vi "AlliGator Calibrate Single Phasor Plot.vi"(0 "Raw Phasor Plot":T6={"Phasor Plot Name"="", "Raw Phasor Plot"=[], "Phasor Frequency"=160000000.0, "[Decay Metadata]"=[], "Raw Phasor Plot SDV"=[], "Phasor SDV Options"={"Compute Estimated SDV"=FALSE, "# Replicas"=100, "Use Estimated Average Phasor"=FALSE}, "[Calibration Phasor]"=[], "Intensity Array"=[]} {"[Decay Metadata]"."# Folds" min=1; "[Decay Metadata]"."ROI Descriptor"."Contours"."Type" items=["No Selection", "Point", "Line", "Rectangle", "Oval", "Polygon", "Freehand Region", "Annulus", "Unused2", "Unused3", "Broken Line", "Freehand Line", "Rotated Rectangle"]}, 5 "Calibration Phasor":T1, 7 "Calibration Phasor Series":T5, 9 "Phasor Calibration Map":T2={"Phasor Frequency"=80000000.0, "Calibration Lifetime"=1e-09, "ROI Centers"=[], "ROI Descriptors"=[], "Map Resolution X"=0, "Map Resolution Y"=0, "z Array"=[]} {"ROI Descriptors"."Contours"."Type" items=["No Selection", "Point", "Line", "Rectangle", "Oval", "Polygon", "Freehand Region", "Annulus", "Unused2", "Unused3", "Broken Line", "Freehand Line", "Rotated Rectangle"]}, 11 "Error In":errorcluster, 12 "Calibration Map MD5 Digest":string, 13 "Phasor Frequency":dbl[unit]) -> (4 "[Calibrated Phasor]":T4[](array[typedef]), 6 "# Recalibrated Phasors":i32, 8 "[Calibration Phasor]":T1[](array[typedef]), 15 "Error Out":errorcluster)   [LabVIEW 2021, in "AlliGator Phasor Calibration.lvlib"]
doc: "Applies phasor calibration to a single phasor plot.\n\nTakes into account whether a single phasor calibration, a phasor map or a phasor calibration series is used.\n\nFor a calibration map, takes into account the location of each individual phasor in the phasor plot."
uses:
  AlliGator Phasor Calibration.lvlib
  Phasor Graph/AlliGator Raw Phasor Plot Data v5.ctl
  Phasor/Phasor (g, s).ctl
  Phasor Graph/AlliGator Decay Metadata v3.ctl
  Decay Analysis/Decay Preprocessing/AlliGator Decay Background Subtraction Info.ctl
  Decay Analysis/Decay Preprocessing/AlliGator Baseline Subtraction Method.ctl
  Graphs/XY Graph/XY Graph Plot Shift Parameters.ctl
  Graphs/XY Graph/XY Graph Plot Shift Method.ctl
  Decay Analysis/Decay Preprocessing/AlliGator Decay Extrapolation Parameters.ctl
  Phasor/Phasor Standard Deviation Options.ctl
  Phasor/Calibration Phasor (m, phi).ctl
  Phasor/Phasor Reference Series.ctl
  Phasor/Phasor Calibration Map v2.ctl
  Settings/AlliGator Settings List.ctl
  Phasor/Phasor Calibration Type.ctl
  Utilities/Utilities.lvlib
  Phasor/Phasor.lvlib
  Settings/AlliGator Settings.lvlib
  Phasor Graph/AlliGator Phasor Graph.lvlib
  Decay Analysis/Decay Preprocessing/AlliGator Decay Preprocessing.lvlib
  Graphs/XY Graph/XY Graph Add-Ons.lvlib
panel:
  # "see the AlliGator License on the block diagram (Ctrl+E or Window:Show Block Diagram)"
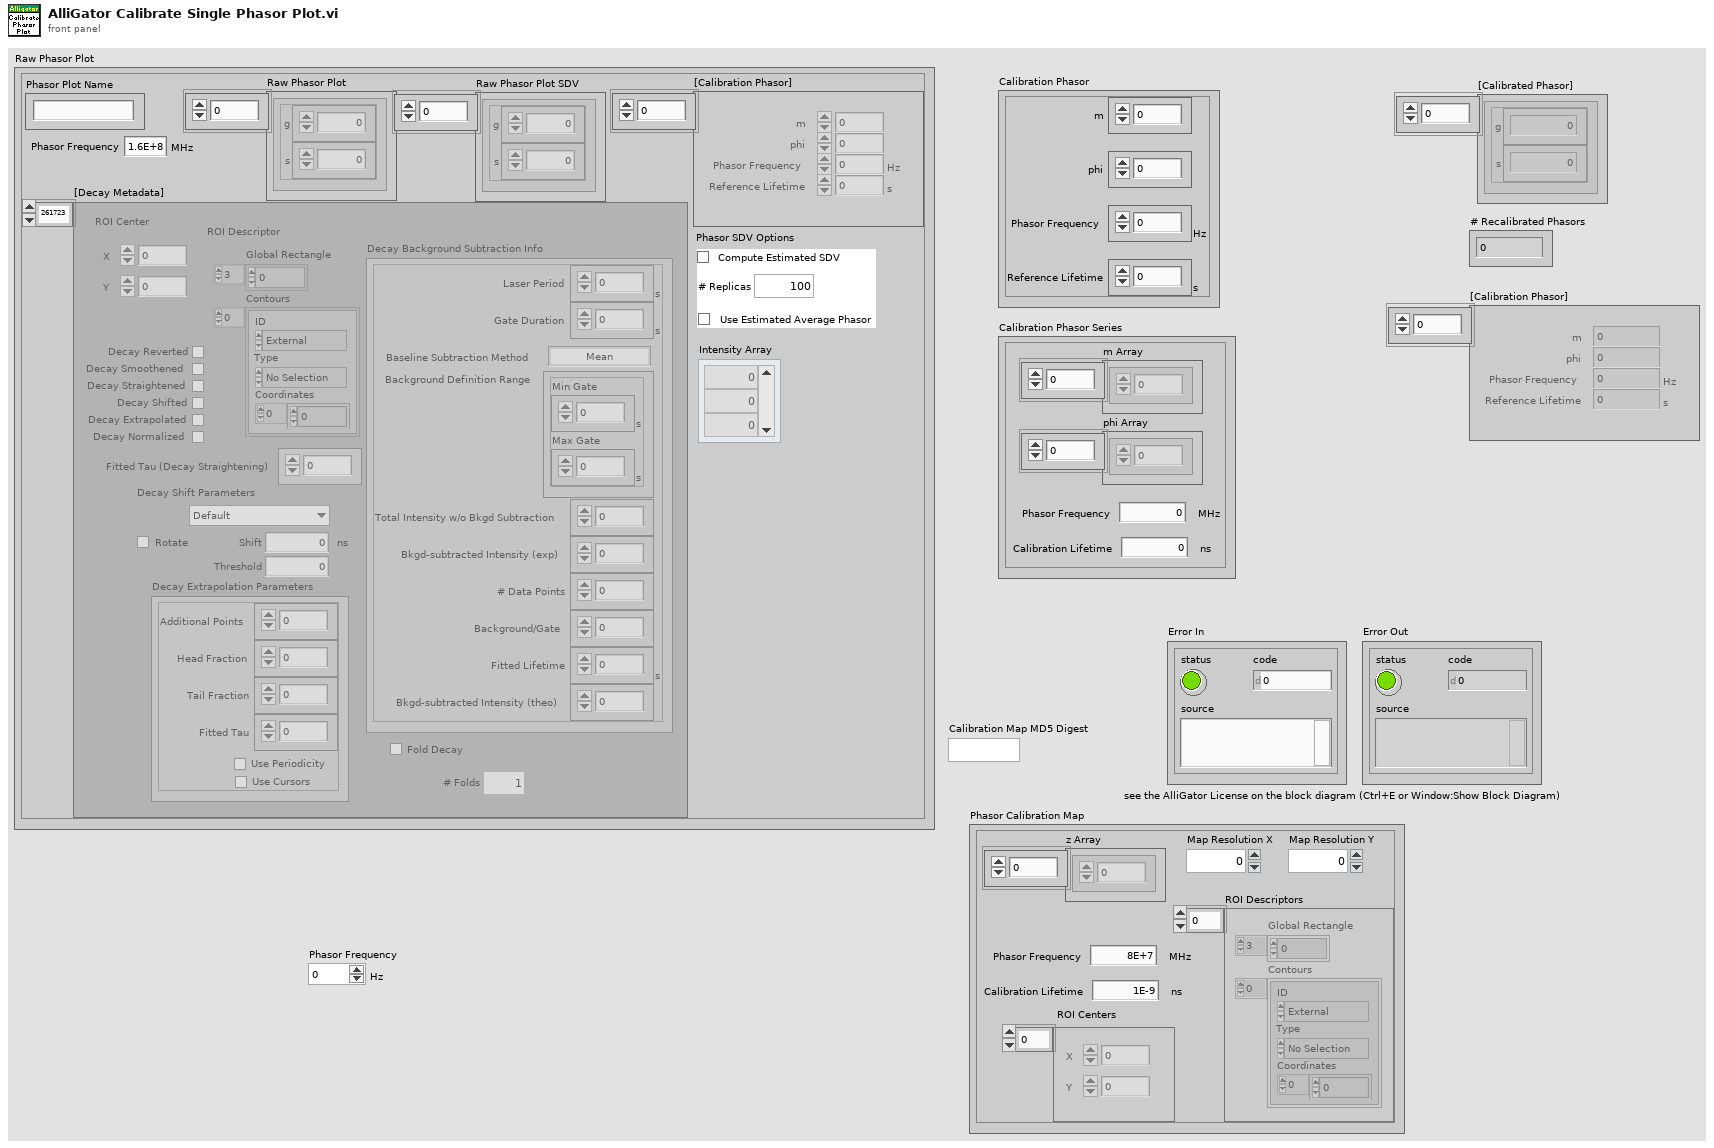
[diagram p1: front panel]
types:
  T1 = typedef "Phasor.lvlib/Calibration Phasor (m, phi).ctl" = cluster{"m":dbl, "phi":dbl, "Phasor Frequency":dbl[unit], "Reference Lifetime":dbl[unit]}
  T2 = typedef "Phasor.lvlib/Phasor Calibration Map v2.ctl" = cluster{"Phasor Frequency":dbl[unit], "Calibration Lifetime":dbl[unit], "ROI Centers":cluster{"X":i32, "Y":i32}[], "ROI Descriptors":T3[], "Map Resolution X":i32, "Map Resolution Y":i32, "z Array":cdb[]}
  T3 = typedef "ROI Descriptor" = cluster{"Global Rectangle":i32[], "Contours":cluster{"ID":enum32{"External", "Internal"}, "Type":u32, "Coordinates":i32[]}[]}
  T4 = typedef "Phasor.lvlib/Phasor (g, s).ctl" = cluster{"g":dbl, "s":dbl}
  T5 = typedef "Phasor.lvlib/Phasor Reference Series.ctl" = cluster{"m Array":dbl[], "phi Array":dbl[], "Phasor Frequency":dbl[unit], "Calibration Lifetime":dbl[unit]}
  T6 = typedef "AlliGator Phasor Graph.lvlib/AlliGator Raw Phasor Plot Data v5.ctl" = cluster{"Phasor Plot Name":string, "Raw Phasor Plot":T4[], "Phasor Frequency":dbl[unit], "[Decay Metadata]":T7[], "Raw Phasor Plot SDV":T4[], "Phasor SDV Options":T13, "[Calibration Phasor]":T1[], "Intensity Array":dbl[]}
  T7 = typedef "AlliGator Phasor Graph.lvlib/AlliGator Decay Metadata v3.ctl" = cluster{"ROI Descriptor":T3, "ROI Center":cluster{"X":i32, "Y":i32}, "Decay Background Subtraction Info":T8, "Decay Reverted":bool, "Decay Smoothened":bool, "Decay Straightened":bool, "Fitted Tau (Decay Straightening)":dbl, "Decay Shift Parameters":T10, "Decay Shifted":bool, "Decay Extrapolated":bool, "Decay Extrapolation Parameters":T12, "Decay Normalized":bool, "Fold Decay":bool, "# Folds":u32}
  T8 = typedef "AlliGator Decay Preprocessing.lvlib/AlliGator Decay Background Subtraction Info.ctl" = cluster{"Laser Period":dbl[unit], "Gate Duration":dbl[unit], "Baseline Subtraction Method":T9, "Background Definition Range":cluster{"Min Gate":dbl[unit], "Max Gate":dbl[unit]}, "Total Intensity w/o Bkgd Subtraction":dbl, "Bkgd-subtracted Intensity (exp)":dbl, "# Data Points":i32, "Background/Gate":dbl, "Fitted Lifetime":dbl[unit], "Bkgd-subtracted Intensity (theo)":dbl}
  T9 = typedef "AlliGator Decay Preprocessing.lvlib/AlliGator Baseline Subtraction Method.ctl" = enum16{"Mean", "Min", "Square Gated Single-Exponential", "File", "Constant"}
  T10 = typedef "XY Graph Add-Ons.lvlib/XY Graph Plot Shift Parameters.ctl" = cluster{"Type":T11, "Shift":dbl[unit], "Threshold":dbl, "Rotate":bool}
  T11 = typedef "XY Graph Add-Ons.lvlib/XY Graph Plot Shift Method.ctl" = enum16{"Default", "CFD", "Threshold", "Cross-Correlation"}
  T12 = typedef "AlliGator Decay Preprocessing.lvlib/AlliGator Decay Extrapolation Parameters.ctl" = cluster{"Additional Points":u32, "Head Fraction":dbl, "Fitted Tau":dbl, "Use Periodicity":bool, "Use Cursors":bool, "Tail Fraction":dbl}
  T13 = typedef "Phasor.lvlib/Phasor Standard Deviation Options.ctl" = cluster{"Compute Estimated SDV":bool, "# Replicas":u32, "Use Estimated Average Phasor":bool}
  T14 = typedef "Phasor.lvlib/Phasor Calibration Type.ctl" = enum16{"None", "Single Phasor", "Phasor Series", "Phasor Map"}
  T15 = typedef "AlliGator Settings.lvlib/AlliGator Settings List.ctl" = enum16{"GUI:Visible Settings Tab", "GUI:Last Run Version", "Source Image:Use Image Histogram for Contrast", "Source Image:Low Count Pixels Rejection Options", "Source Image:High Count Pixels Rejection Options", "Source Image:Use Image Brightness", "Source Image:Blend Overlay with Image Background", "Source Image:Use Fixed ROI Diameter", "Source Image:ROI Diameter", "Source Image:ROI Center Color", "Source Image:Peak Threshold", "Source Image:Intensity Threshold", "Source Image:Image Binning Options", "Source Image:Image Smoothing Options", "Source Image:Image Histogram Active", "Source Image:Invert Binary Mask", "Source Image:Hot Pixel Removal", "Source Image:Overlay Analyzed ROI Center", "Source Image:Auto-Adjust Contrast", "Source Image:Histogram Lower Percentile", "Source Image:Histogram Upper Percentile", "Source Image:Save Source Image", "Source Image:Scale Bar Options", "Source Image:Image Resolution (Pixel Size)", "Source Image:Flatfield Correction", "Source Image:Show Dead Left Columns Correction", "Source Image:Dead Left Columns Correction", "Source Image:Image Pre-Processing Operations Order", "Source Image:Overlay ROI Median", "Source Image:Median Overlay Color", "Data Information:Gate Width", "Data Information:Nanotime Gate Separation", "Data Information:Macrotime Gate Separation", "Data Information:Gate Step", "Data Information:# Gates", "Data Information:Gate Image Exposure", "Data Information:Gate Image Integration", "Data Information:Gates to Skip", "Data Information:Gates to Keep", "Data Information:Define Gates to", "Data Information:Channel Name", "Data Information:Available Channel Names", "Data Information:Channel Arithmetic", "Data Information:Background File Subtraction", "Data Information:Background File", "Data Information:Background Scaling Factor", "Data Information:Background Pile-up Correction", "Data Information:Background Pixel Well Capacity", "Data Information:Laser Period", "Data Information:SYNC Period", "Data Information:Pile-up Correction", "Data Information:Pixel Well Capacity", "Data Information:Dataset Scaling Factor", "Fluorescence Decay_Decay Pre-Processing:Reverse Gates", "Fluorescence Decay_Decay Pre-Processing:Verbose Decay Pre-Processing", "Fluorescence Decay_Decay Pre-Processing:Use Decay Pre-Processing", "Fluorescence Decay_Decay Pre-Processing:Background Subtraction", "Fluorescence Decay_Decay Pre-Processing:Background Definition Range", "Fluorescence Decay_Decay Pre-Processing:Baseline Subtraction Method", "Fluorescence Decay_Decay Pre-Processing:Decay Pre-Processing Operations Order", "Fluorescence Decay_Decay Pre-Processing:Smoothing Parameter", "Fluorescence Decay_Decay Pre-Processing:Shift Decay", "Fluorescence Decay_Decay Pre-Processing:Decay Shift Parameters", "Fluorescence Decay_Decay Pre-Processing:Fold Decay", "Fluorescence Decay_Decay Pre-Processing:# Folds", "Fluorescence Decay_Decay Pre-Processing:1-Normalize Decay", "Fluorescence Decay_Decay Pre-Processing:[0-1]-Normalize Decay", "Fluorescence Decay_Decay Pre-Processing:Smoothen Decay", "Fluorescence Decay_Decay Pre-Processing:Extrapolate Decay", "Fluorescence Decay_Decay Pre-Processing:Use Periodicity", "Fluorescence Decay_Decay Pre-Processing:Use Cursors", "Fluorescence Decay_Decay Pre-Processing:Tail Fraction", "Fluorescence Decay_Decay Pre-Processing:Head Fraction", "Fluorescence Decay_Decay Pre-Processing:Additional Points", "Fluorescence Decay_Decay Pre-Processing:Straighten Decay", "Fluorescence Decay_Decay Pre-Processing:Constant Background", "Fluorescence Decay_Decay Pre-Processing:Pixel-Normalize Decay", "Fluorescence Decay_Advanced Analysis:Extract IRF instead of Decay", "Fluorescence Decay_Advanced Analysis:IRF Extraction Options", "Fluorescence Decay_Advanced Analysis:IRF Optimization Options", "Fluorescence Decay_Advanced Analysis:Square Pulse Options", "Fluorescence Decay_Advanced Analysis:IRF Order", "Fluorescence Decay_Advanced Analysis:IRF Time Constants", "Fluorescence Decay_Advanced Analysis:Wavelet Analysis Options", "Fluorescence Decay_Advanced Analysis:Average Lifetime Options", "Fluorescence Decay_Fit Options:Fit Options", "Fluorescence Decay_Fit Options:Use Legacy Fitting Approach", "Fluorescence Decay_Fit Options:Use Data Information Laser Period", "Fluorescence Decay_Fit Parameters:Displayed Fit Parameters", "Fluorescence Decay_Fit Parameters:Fit Parameter Constraints", "Fluorescence Decay_Fit Parameters:Export Tabulated Results", "Fluorescence Decay_Fit Parameters:MLE Baseline Offset Type", "Fluorescence Decay_Fit Parameters:MLE Baseline Offset", "Fluorescence Decay_Fit Parameters:Guess Parameter Names", "Fluorescence Decay_Fit Parameters:Guess Parameter Values", "Fluorescence Decay_Fit Parameters:Guess Parameters Options", "Fluorescence Decay_Fit Parameters:Optimal Offset Selection Criterion", "Fluorescence Decay_Styles:Show Last Decay Only", "Fluorescence Decay_Styles:Decay Graph Color Array", "Fluorescence Decay:Decay Graph Active", "Fluorescence Decay Statistics:Min Peak Value", "Fluorescence Decay Statistics:Reject Low Decay Peak Pixels", "Fluorescence Decay Statistics:Reject High Decay Peak Pixels", "Fluorescence Decay Statistics:Max Peak Value", "Time Traces:Use File Timestamp", "Time Traces:Time Step", "Time Traces:Use Intensity Correction File", "Time Traces:Intensity Correction File", "Phasor Plot:Phasor Plot Smoothing Options", "Phasor Plot:Phasor Plot Size", "Phasor Plot:Phasor Plot Graphics Options", "Phasor Plot:Cumulative Phasor Plot", "Phasor Plot:Use Phasor Brightness", "Phasor Plot:Blend Overlay with Phasor Background", "Phasor Plot:Save Phasor Plot", "Phasor Plot:Show References", "Phasor Plot:Phasor Ratio Decay Range", "Phasor Plot:Exponential Fading", "Phasor Plot:Phasor Ratio Reference Colors", "Phasor Plot:Reference Radius", "Phasor Plot:Show Color Map Vertices", "Phasor Plot:Phasor Plot Active", "Phasor Plot:Phasor Ratio Color Map Type", "Phasor Plot:Phasor Ratio Color Map", "Phasor Plot:Phasor Ratio Display Range", "Phasor Plot:Selected Image ROI(s)", "Phasor Plot:All Image ROIs", "Phasor Plot:Selected Phasor Plot ROI(s)", "Phasor Plot:All Phasor Plot ROIs", "Phasor Plot:Phasor Ratio Color-Coded Quantity", "Phasor Plot:Store Phasor Harmonics", "Phasor Plot:Draw Reference Segment", "Phasor Plot:User-Defined Quantity", "Phasor Plot:Color Scale High Color", "Phasor Plot:Color Scale Low Color", "Phasor Plot:Intensity-weighted Phasor Plot", "Phasor Graph:Phasor Frequency", "Phasor Graph:Phasor Ratio Type", "Phasor Graph:Pixel-level Phasor Computation", "Phasor Graph:Save Phasor Graph", "Phasor Graph:Phasor Graph Active", "Phasor Graph:Phasor SDV Options", "Phasor Graph:Intensity-weighted Phasor Graph", "Phasor Graph:Define Shortest Lifetime as", "Phasor Calibration:Use Backup Calibration if needed", "Phasor Calibration:Backup Calibration Type", "Phasor Calibration:Calibration Type", "Phasor Calibration:Calibration Lifetime", "Phasor Calibration:Calibration Map Algorithm", "Single-Exponential Phasor Locus (SEPL):Gate Parameters", "Single-Exponential Phasor Locus (SEPL):User-defined Gate", "Single-Exponential Phasor Locus (SEPL):User-defined IRF", "Single-Exponential Phasor Locus (SEPL):Phasor Parameters", "Single-Exponential Phasor Locus (SEPL):Decay & IRF Parameters", "Single-Exponential Phasor Locus (SEPL):Display Parameters", "Lifetime Analysis:Decay Analysis Parameters", "Lifetime Analysis:Lifetime Map Active", "Plugins:Python Settings", "Miscellaneous:Verbose Mode", "Miscellaneous:Beep after Script", "Miscellaneous:Saved Image File Format", "Miscellaneous:Exported Gate Image Settings", "Miscellaneous:Include Loading in Timing", "Miscellaneous:Verbose Settings Mode", "Miscellaneous:Histogram Options", "Miscellaneous:Beep on Error", "Miscellaneous:# Logical Processors Used", "Miscellaneous:ROI Description Max Characters", "Miscellaneous:Verbose Error Mode", "Miscellaneous:Transparent Mask Color"}
  T16 = cluster{"Use Backup Calibration if needed?":bool, "Calibration Type":T14}
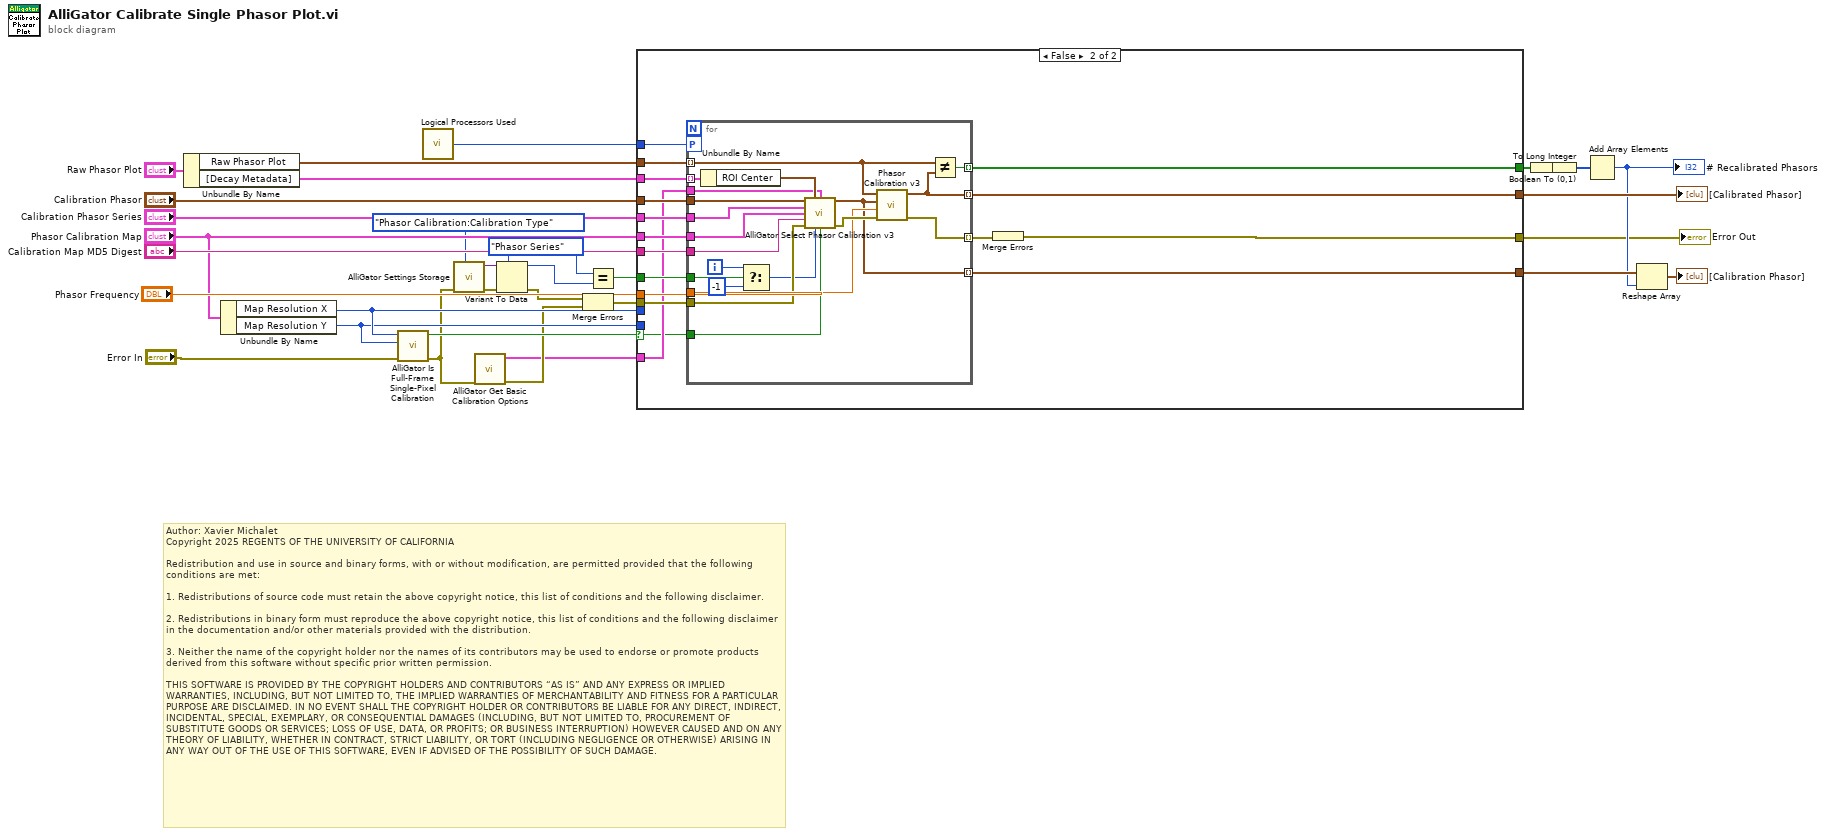
[diagram p0: block diagram]
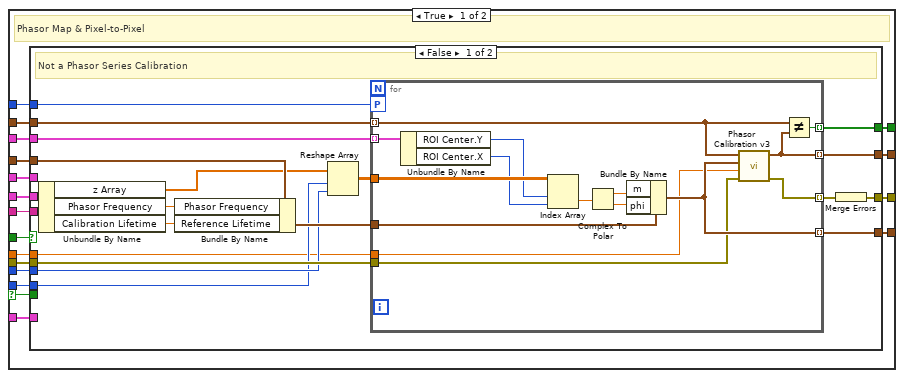
[diagram p2: hidden frame]
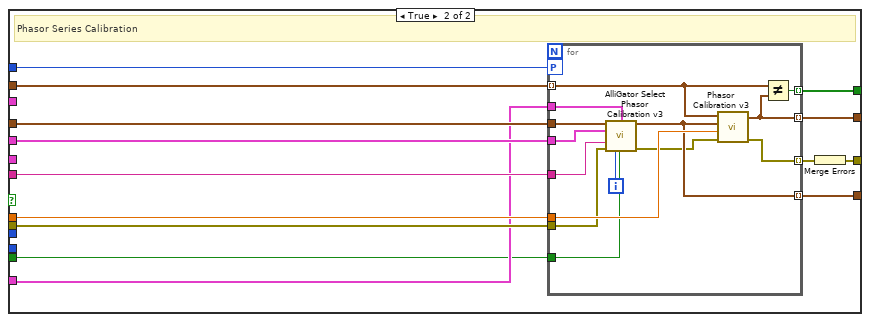
[diagram p3: hidden frame]
diagram:
  w6 = Phasor_Calibration_Type."Phasor Series" ("Calibration Type")
  # "Author: Xavier Michalet\nCopyright 2025 REGENTS OF THE UNIVERSITY OF CALIFORNIA\n\nRedistribution and use in source and binary forms, with or without modification, are permitted provided that the following conditions are met:\n\n1. Redistributions of source code must retain the above copyright notice, this list of conditions and the following disclaimer.\n\n2. Redistributions in binary form must reproduce the above copyright notice, this list of conditions and the following disclaimer in the documentation and/or other materials provided with the distribution.\n\n3. Neither the name of the copyright holder nor the names of its contributors may be used to endorse or promote products derived from this software without specific prior written permission.\n\nTHIS SOFTWARE IS PROVIDED BY THE COPYRIGHT HOLDERS AND CONTRIBUTORS “AS IS” AND ANY EXPRESS OR IMPLIED WARRANTIES, INCLUDING, BUT NOT LIMITED TO, THE IMPLIED WARRANTIES OF MERCHANTABILITY AND FITNESS FOR A PARTICULAR PURPOSE ARE DISCLAIMED. IN NO EVENT SHALL THE COPYRIGHT HOLDER OR CONTRIBUTORS BE LIABLE FOR ANY DIRECT, INDIRECT, INCIDENTAL, SPECIAL, EXEMPLARY, OR CONSEQUENTIAL DAMAGES (INCLUDING, BUT NOT LIMITED TO, PROCUREMENT OF SUBSTITUTE GOODS OR SERVICES; LOSS OF USE, DATA, OR PROFITS; OR BUSINESS INTERRUPTION) HOWEVER CAUSED AND ON ANY THEORY OF LIABILITY, WHETHER IN CONTRACT, STRICT LIABILITY, OR TORT (INCLUDING NEGLIGENCE OR OTHERWISE) ARISING IN ANY WAY OUT OF THE USE OF THIS SOFTWARE, EVEN IF ADVISED OF THE POSSIBILITY OF SUCH DAMAGE."
  n1 = Unbundle By Name("Raw Phasor Plot") -> ("Raw Phasor Plot"=w28:T4[], "[Decay Metadata]"=w27:T7[])
  n2 = Unbundle By Name("Phasor Calibration Map") -> ("Map Resolution X"=w17:i32, "Map Resolution Y"=w14:i32)
  n3 = call "AlliGator Is Full-Frame Single-Pixel Calibration.vi"("error in (no error)"="Error In", "Map Resolution Y"=w14, "Map Resolution X"=w17) -> ("error out"=w3:errorcluster, "Full-Frame Single-Pixel Calibration?"=w15:bool)  [unwired: 7 in]
  n4 = call "Logical Processors Used.vi"() -> ("# Logical Processor Used"=w13:i32)  [unwired: 6 in]
  n5 = call "AlliGator Settings Storage.vi"("AlliGator Settings List"=AlliGator_Settings_List."Phasor Calibration:Calibration Type", "Error In"=w3) -> ("Error Out"=w9:errorcluster, "Variant Data out"=w10:variant)  [unwired: 8 in]
  n6 = call "AlliGator Get Basic Calibration Options.vi"("error in (no error)"=w3) -> ("error out"=w2:errorcluster, "Basic Calibration Options"=w1:T16)  [unwired: 9 in]
  n7 = Variant To Data(error in=w9, type=w6, Variant=w10) -> (data=w7:T14, error out=w8:errorcluster)
  n8 = Merge Errors(w8, w2) -> (w4:errorcluster)
  n9 = Equal?(x=w6, y=w7) -> (x = y?=w5:bool)
  n10 = case shown="False" w15 {
    selector: w15 -> [w33 w113]
    tunnel: "Calibration Phasor" -> [w44 w129]
    tunnel: "Calibration Phasor Series" -> [w36 w128]
    tunnel: [w50 w127] -> w29
    tunnel: w28 -> [w49 w126]
    tunnel: "Phasor Calibration Map" -> [w48 w125]
    tunnel: w27 -> [w47 w124]
    tunnel: "Calibration Map MD5 Digest" -> [w35 w123]
    tunnel: [w46 w122] -> w25
    tunnel: "Phasor Frequency" -> [w38 w121]
    tunnel: [w45 w120] -> w21
    tunnel: w4 -> [w43 w119]
    tunnel: w17 -> [w42 _]
    tunnel: w14 -> [w41 _]
    tunnel: w13 -> [w40 w118]
    tunnel: [w39 w116] -> w12
    tunnel: w5 -> [w37 w115]
    tunnel: w1 -> [w34 w114]
    frame True {
      # "Phasor Map & Pixel-to-Pixel"
      n11 = case shown="False" w37 {
        tunnel: [w69 w98] -> w50
        tunnel: w49 -> [w68 w97]
        tunnel: w48 -> [w67 _]
        tunnel: w47 -> [w66 _]
        tunnel: [w65 w96] -> w46
        tunnel: [w64 w95] -> w45
        tunnel: w44 -> [w63 w88]
        tunnel: w43 -> [w60 w94]
        tunnel: w42 -> [w58 _]
        tunnel: w41 -> [w57 _]
        tunnel: w40 -> [w54 w93]
        tunnel: [w52 w91] -> w39
        tunnel: w38 -> [w51 w90]
        tunnel: w36 -> [_ w89]
        tunnel: w35 -> [_ w87]
        tunnel: w34 -> [_ w86]
        tunnel: w33 -> [_ w85]
        frame False {
          # "Not a Phasor Series Calibration"
          n12 = Unbundle By Name(w67) -> ("z Array"=w59:cdb[], "Phasor Frequency"=w55:dbl[unit], "Calibration Lifetime"=w61:dbl[unit])
          n13 = Bundle By Name(cluster=w63, "Phasor Frequency"=w55, "Reference Lifetime"=w61) -> (w62:T1)
          n14 = Reshape Array(w59, w57, w58) -> (w56:cdb[][])
          n15 = for {
            tunnel: w68 -> [w83] mode=indexing
            tunnel: [w82] -> w69 mode=indexing
            tunnel: w66 -> [w84] mode=indexing
            tunnel: [w80] -> w53 mode=indexing
            workers-P: w54 -> [_]
            tunnel: [w81] -> w65 mode=indexing
            tunnel: [w78] -> w64 mode=indexing
            tunnel: w62 -> [w79]
            tunnel: w51 -> [w77]
            tunnel: w56 -> [w76]
            tunnel: w60 -> [w74]
            n16 = Unbundle By Name(w84) -> ("ROI Center.Y"=w73:i32, "ROI Center.X"=w72:i32)
            n17 = Index Array(array=w76, index (row)=w73, index (col)=w72) -> (element=w75:cdb)
            n18 = Complex To Polar(r * e^(i*theta)=w75) -> (r=w71:dbl, theta=w70:dbl)
            n19 = Bundle By Name(cluster=w79, "m"=w71, "phi"=w70) -> (w78:T1)
            n20 = call "Phasor Calibration v3.vi"("Error In"=w74, "Phasor Frequency"=w77, "Calibration Phasor"=w78, "Measured Phasor"=w83) -> ("Error Out"=w80:errorcluster, "Calibrated Phasor"=w82:T4)  [unwired: 2 in, 4 out]
            n21 = Not Equal?(x=w83, y=w82) -> (x != y?=w81:bool)
          }
          n22 = Merge Errors(w53) -> (w52:errorcluster)
        }
        frame True {
          # "Phasor Series Calibration"
          n23 = for {
            tunnel: w97 -> [w112] mode=indexing
            tunnel: [w111] -> w98 mode=indexing
            tunnel: [w109] -> w92 mode=indexing
            workers-P: w93 -> [_]
            tunnel: [w110] -> w96 mode=indexing
            tunnel: [w103] -> w95 mode=indexing
            tunnel: w90 -> [w108]
            tunnel: w94 -> [w102]
            tunnel: w89 -> [w107]
            tunnel: w88 -> [w106]
            tunnel: w87 -> [w104]
            tunnel: w86 -> [w100]
            tunnel: w85 -> [w99]
            i -> [w105]
            n24 = call "AlliGator Select Phasor Calibration v3.vi"("Calibration Phasor"=w106, "Basic Calibration Options"=w100, "Calibration Phasor Series"=w107, "Calibration Map MD5 Digest"=w104, "Error In"=w102, "Current Data Set (-1: single)"=w105, "Full-Frame Single-Pixel Calibration?"=w99) -> ("Calibration Phasor"=w103:T1, "Error Out"=w101:errorcluster)  [unwired: 6 in, 1 out]
            n25 = call "Phasor Calibration v3.vi"("Error In"=w101, "Phasor Frequency"=w108, "Calibration Phasor"=w103, "Measured Phasor"=w112) -> ("Error Out"=w109:errorcluster, "Calibrated Phasor"=w111:T4)  [unwired: 2 in, 4 out]
            n26 = Not Equal?(x=w112, y=w111) -> (x != y?=w110:bool)
          }
          n27 = Merge Errors(w92) -> (w91:errorcluster)
        }
      }
    }
    frame False {
      n28 = for {
        tunnel: w126 -> [w142] mode=indexing
        tunnel: w128 -> [w147]
        tunnel: w129 -> [w148]
        tunnel: [w141] -> w127 mode=indexing
        tunnel: w125 -> [w146]
        tunnel: w124 -> [w145] mode=indexing
        tunnel: w119 -> [w149]
        tunnel: [w138] -> w117 mode=indexing
        workers-P: w118 -> [_]
        tunnel: w123 -> [w143]
        tunnel: [w140] -> w122 mode=indexing
        tunnel: w121 -> [w137]
        tunnel: [w136] -> w120 mode=indexing
        tunnel: w115 -> [w132]
        tunnel: w114 -> [w131]
        tunnel: w113 -> [w130]
        i -> [w135]
        n29 = Unbundle By Name(w145) -> ("ROI Center"=w144:cluster{"X":i32, "Y":i32})
        n30 = Select(t=w135, s=w132, f=-1) -> (s? t:f=w134:i32)
        n31 = call "AlliGator Select Phasor Calibration v3.vi"("Calibration Phasor"=w148, "ROI Center (Default: undefined)"=w144, "Basic Calibration Options"=w131, "Calibration Phasor Series"=w147, "Phasor Calibration Map"=w146, "Calibration Map MD5 Digest"=w143, "Error In"=w149, "Current Data Set (-1: single)"=w134, "Full-Frame Single-Pixel Calibration?"=w130) -> ("Calibration Phasor"=w136:T1, "Error Out"=w139:errorcluster)  [unwired: 4 in, 1 out]
        n32 = call "Phasor Calibration v3.vi"("Error In"=w139, "Phasor Frequency"=w137, "Calibration Phasor"=w136, "Measured Phasor"=w142) -> ("Error Out"=w138:errorcluster, "Calibrated Phasor"=w141:T4)  [unwired: 2 in, 4 out]
        n33 = Not Equal?(x=w142, y=w141) -> (x != y?=w140:bool)
      }
      n34 = Merge Errors(w117) -> (w116:errorcluster)
    }
  }
  "Error Out" <- w12
  "[Calibrated Phasor]" <- w29
  n35 = Boolean To (0,1)(Boolean=w25) -> (0, 1=w24:i16[])
  n36 = To Long Integer(number=w24) -> (32bit integer=w23:i32[])
  n37 = Add Array Elements(numeric array=w23) -> (sum=w20:i32)
  "# Recalibrated Phasors" <- w20
  n38 = Reshape Array(w21, w20) -> (→"[Calibration Phasor]":T1[])
